vi "Calcul itératif.vi"(8 "error in (no error)":T1 caption="entrée d'erreur (pas d'erreur)", 10 "Température capteur 1-2-3-4-Ambiant":dbl[](array[numeric]), 11 "Position des capteurs":dbl[][](array[numeric])) -> (0 "error out":T1 caption="sortie d'erreur", 3 "DATA - T/R1/R2/R3":dbl[](array[numeric]) format="%#_13g")   [LabVIEW 2018]
panel:
  in  "T max":dbl
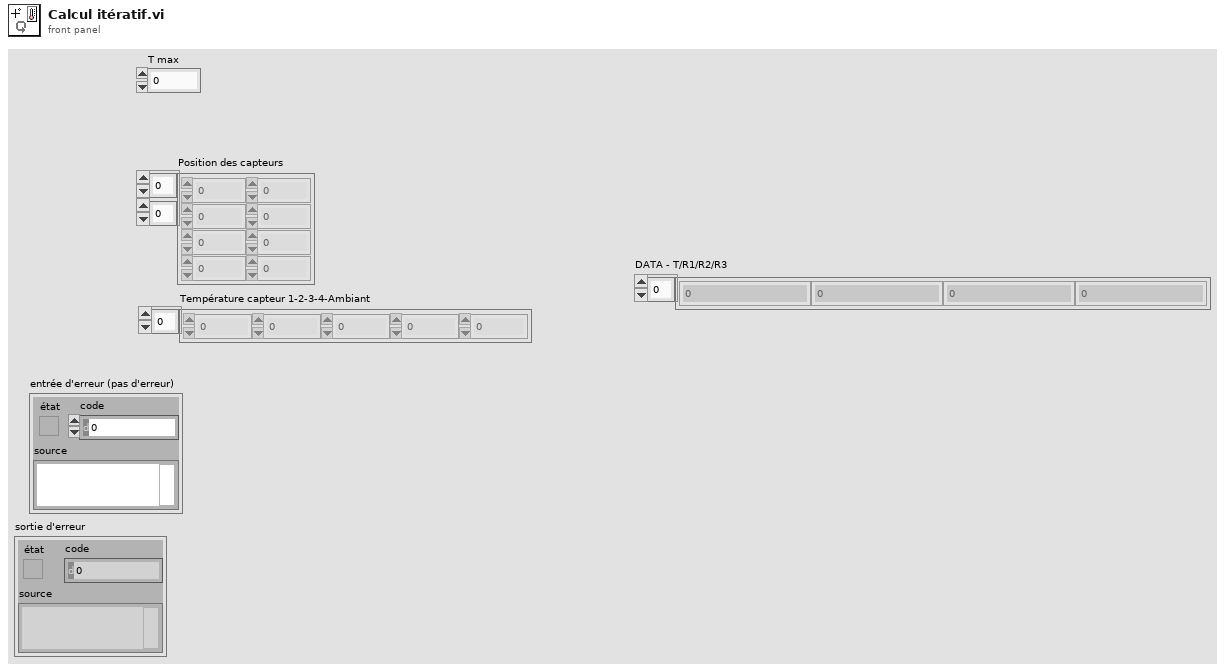
[diagram p1: front panel]
types:
  T1 = cluster{"état":bool, "code":i32, "source":string}
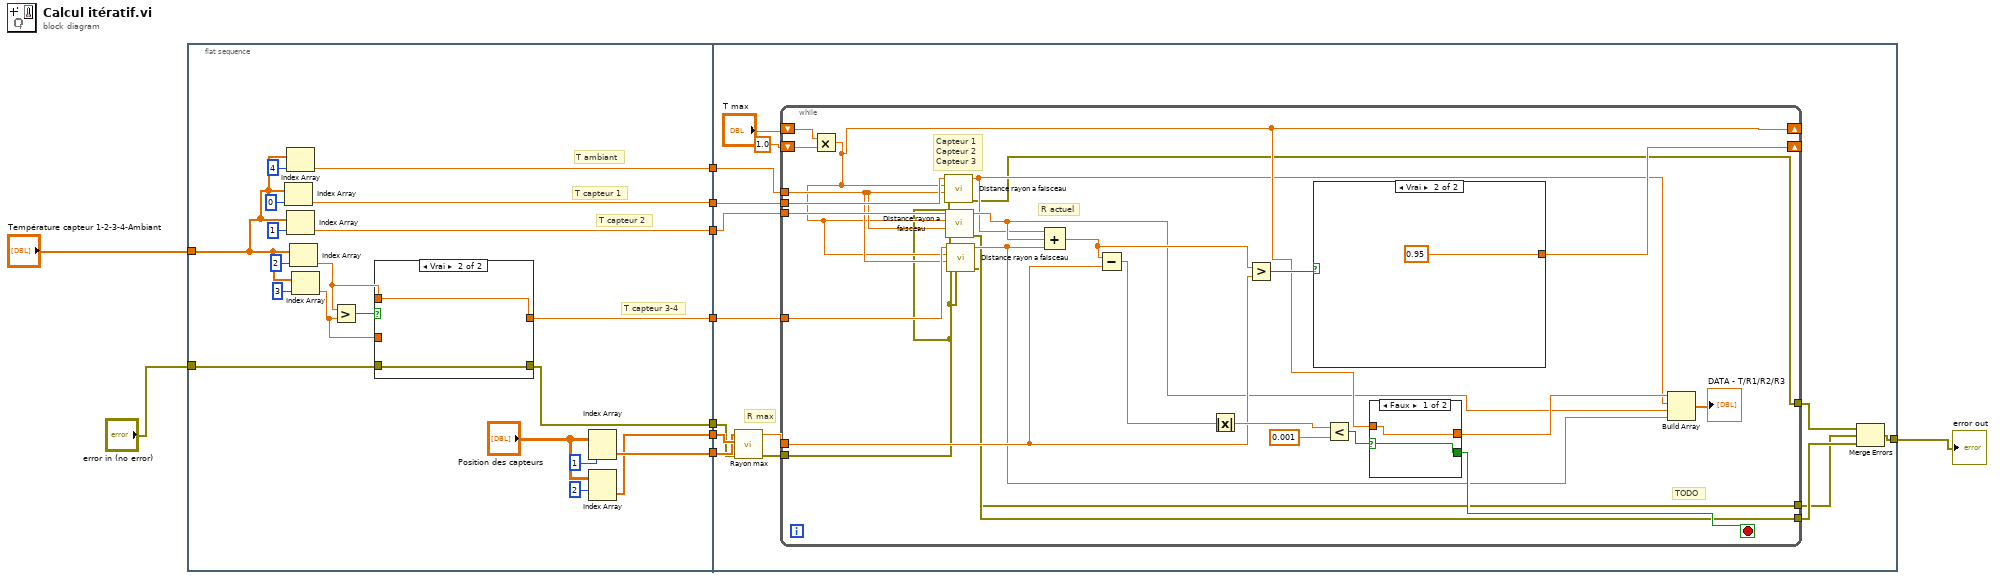
[diagram p0: block diagram]
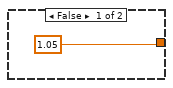
[diagram p4: hidden frame]
diagram:
  n1 = flat-sequence {
    tunnel: "Température capteur 1-2-3-4-Ambiant" -> [w20]
    tunnel: [w26] -> w10
    tunnel: [w22] -> w9
    tunnel: [w21] -> w8
    tunnel: [w18] -> w7
    tunnel: [w14] -> w5
    tunnel: [w13] -> w4
    tunnel: "error in (no error)" -> [w12]
    tunnel: [w11] -> w2
    tunnel: w10 -> [w46]
    tunnel: w9 -> [w49]
    tunnel: w8 -> [w47]
    tunnel: w7 -> [w48]
    tunnel: w5 -> [w42]
    tunnel: w4 -> [w43]
    tunnel: w2 -> [w40]
    tunnel: [w35] -> w1
    frame #0 {
      # "T capteur 3-4"
      # "T capteur 2"
      # "T capteur 1"
      # "T ambiant"
      n2 = Index Array(array=w20, index=0 ("indice")) -> (element=w22:dbl)
      n3 = Index Array(array=w20, index=4 ("indice")) -> (element=w18:dbl)
      n4 = Index Array(array=w20, index=1 ("indice")) -> (element=w21:dbl)
      n5 = Index Array(array=w20, index=2 ("indice")) -> (element=w27:dbl)
      n6 = Index Array(array=w20, index=3 ("indice")) -> (element=w25:dbl)
      n7 = Greater?(x=w27, y=w25) -> (0:w28:bool)
      n8 = case shown="Vrai" w28 {
        tunnel: [w32 w34] -> w26
        tunnel: w27 -> [_ w34]
        tunnel: w25 -> [w32 _]
        tunnel: w12 -> [w31 w33]
        tunnel: [w31 w33] -> w11
        frame False {
        }
        frame True {
        }
      }
      n9 = Index Array(array="Position des capteurs", index (row)=1 ("indice (ligne)")) -> (element=w14:dbl[])  [unwired: 1 in]
      n10 = Index Array(array="Position des capteurs", index (row)=2 ("indice (ligne)")) -> (element=w13:dbl[])  [unwired: 1 in]
    }
    frame #1 {
      # "R max"
      n11 = call "Rayon max.vi"("error in (no error)"=w40, "Capteur 3 ou 4"=w43, "Capteur 2"=w42) -> ("error out"=w39:T1, "Rayon max"=w41:dbl)  [unwired: 7 in]
      n12 = while {
        tunnel: w49 -> [w74]
        tunnel: w48 -> [w71]
        tunnel: w47 -> [w73]
        tunnel: w46 -> [w72]
        shift-right: [w68] -> _
        shift-left: 1.0 -> [w62]
        shift-right: [w59] -> _
        shift-left: "T max" -> [w61]
        tunnel: w41 -> [w60]
        tunnel: w39 -> [w53]
        tunnel: [w52] -> w36
        tunnel: [w51] -> w38
        tunnel: [w50] -> w37
        stop <- w66 stop-if-true
        # "Capteur 1\nCapteur 2\nCapteur 3"
        # "R actuel"
        # "TODO"
        n13 = Multiply(x=w61, y=w62) -> (x*y=w59:dbl)
        n14 = call "Distance rayon a faisceau.vi"("error in (no error)"=w53, "T ambiant"=w71, "T max"=w59, "T capteur"=w74) -> ("error out"=w52:T1, "Rayon"=w54:dbl)  [unwired: 6 in]
        n15 = call "Distance rayon a faisceau.vi"("error in (no error)"=w53, "T ambiant"=w71, "T max"=w59, "T capteur"=w73) -> ("error out"=w51:T1, "Rayon"=w57:dbl)  [unwired: 6 in]
        n16 = call "Distance rayon a faisceau.vi"("error in (no error)"=w53, "T ambiant"=w71, "T max"=w59, "T capteur"=w72) -> ("error out"=w50:T1, "Rayon"=w56:dbl)  [unwired: 6 in]
        n17 = Compound Arithmetic op=ADD(w54, w57, w56) -> (w69:dbl)
        n18 = Subtract(x=w69, y=w60) -> (x-y=w70:dbl)
        n19 = Absolute Value(x=w70) -> (abs(x)=w64:dbl)
        n20 = Greater?(x=w69, y=w60) -> (0:w67:bool)
        n21 = case shown="Vrai" w67 {
          tunnel: [1.05 0.95] -> w68
          frame False {
          }
          frame True {
          }
        }
        n22 = Less?(x=w64, y=0.001) -> (x < y?=w63:bool)
        n23 = case shown="Faux" w63 {
          selector: w63 -> [w76 w78]
          tunnel: [w76 w78] -> w66
          tunnel: w59 -> [w75 w77]
          tunnel: [w75 w77] -> w58
          frame False {
          }
          frame True {
          }
        }
        n24 = Build Array(w58, w54, w57, w56) -> (→"DATA - T/R1/R2/R3":dbl[])
      }
      n25 = Merge Errors(w36, w37, w38) -> (w35:errorcluster)
    }
  }
  "error out" <- w1
